vi "HeaderAction.vi"(0 "InstrClass":refnum<class "Agilent34410A.lvclass"> caption="DNL_LabVIEW Object in", 11 "error in (no error)":errorcluster caption="entrée d'erreur (pas d'erreur)") -> (4 "InstrClassOut":refnum<class "Agilent34410A.lvclass"> caption="DNL_LabVIEW Object out", 6 "DataNames":string[](array[string]), 8 "Instr Name":string, 10 "HeaderString":string, 13 "ArrDatNames":string[](array[string]), 14 "DisplayNames":string[](array[string]), 15 "error out":errorcluster caption="sortie d'erreur")   [LabVIEW 2019, in "Agilent34410A.lvclass"]
uses:
  Agilent34410A.lvclass
  C:/Programmes Labview/LabScanV1A/DevicesClass/BaseDevice/BaseDevice.lvclass
  Agilent34410A.lvclass/Agilent34410A.ctl
  BaseDevice/BaseDevice.lvclass
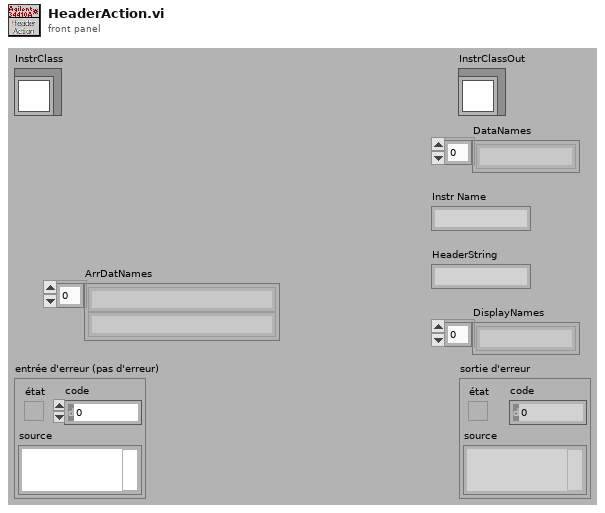
[diagram p1: front panel]
types:
  T1 = typedef "Agilent34410A.lvclass/Agilent34410A_Func.ctl" = enum16{"Read Function (Arb)", "Read Voltage (V)", "Read Current (A)", "Read 2W Resistance (Ohms)", "Read 4W Resistance (Ohms)"}
  T2 = typedef "Agilent34410A DMM_Func.ctl" = enum16{"Capacitance", "Continuity", "Current AC", "Current", "Diode", "Frequency", "4W Resistance", "Period", "Resistance", "Temperature", "Voltage AC", "Voltage"}
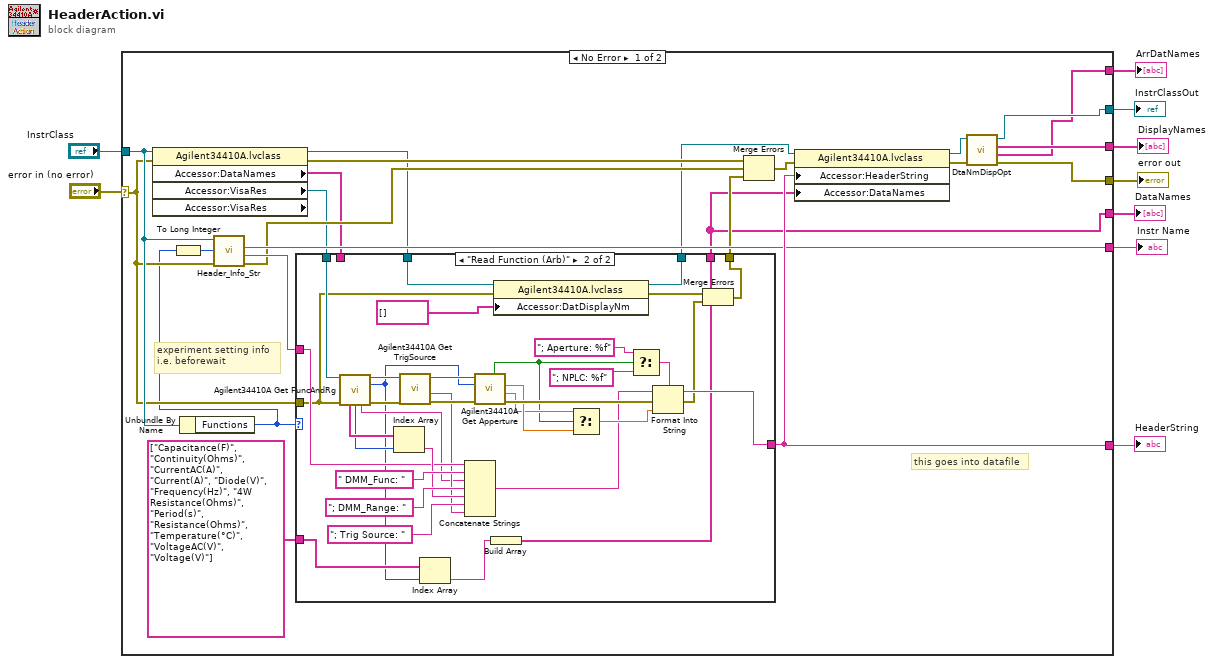
[diagram p0: block diagram]
diagram:
  n1 = case shown="No Error" "error in (no error)" {
    selector: "error in (no error)" -> [w21 w72]
    tunnel: [w31 _] -> w8
    tunnel: [w17 _] -> w7
    tunnel: "InstrClass" -> [w27 w73]
    tunnel: [w10 w72] -> w5
    tunnel: [w12 w73] -> w3
    tunnel: [w26 _] -> w4
    tunnel: [w28 _] -> w2
    tunnel: [w11 _] -> w1
    frame No Error {
      # "this goes into datafile"
      # "experiment setting info\ni.e. beforewait"
      n2 = property class="Agilent34410A.lvclass" props=["Accessor:DataNames", "Accessor:VisaRes", "Accessor:VisaRes"](reference=w27, error in=w21) -> (reference out=w16:refnum<class "Agilent34410A.lvclass">, error out=w32:errorcluster, "Accessor:DataNames"=w19:string[], "Accessor:VisaRes"=w22:refnum<visa-resource-name>)  [unwired: 1 out]
      n3 = Unbundle By Name(w27) -> ("Functions"=w13:T1)
      n4 = To Long Integer(number=w13) -> (32bit integer=w14:i32)
      n5 = call-dynamic "Header_Info_Str.vi"("error in (no error)"=w21, "Functions"=w14, "DefaultDev in"=w27) -> ("error out"=w23:errorcluster, "HdrInfoStr"=w25:string, "InstrumentName"=w26:string)  [unwired: 5 in, 1 out]
      n6 = case shown="\"Read Function (Arb)\"" w13 {
        tunnel: [w36 w50] -> w31
        tunnel: w25 -> [w36 w54]
        tunnel: w22 -> [_ w71]
        tunnel: w21 -> [w35 w42]
        tunnel: [w35 w39] -> w20
        tunnel: w19 -> [w34 _]
        tunnel: [w34 w38] -> w17
        tunnel: string[] ["Capacitance(F)", "Continuity(Ohms)", "CurrentAC(A)", "Current(A)", "Diode(V)", "Frequency(Hz)", "4W Resistance(Ohms)", "Period(s)", "Resistance(Ohms)", "Temperature(°C)", "VoltageAC(V)", "Voltage(V)"] ("Chaînes []") -> [_ w47]
        tunnel: w16 -> [w33 w44]
        tunnel: [w33 w43] -> w15
        frame Default {
        }
        frame "Read Function (Arb)" {
          n7 = call <userlib>:"Agilent34410A Get FuncAndRg.vi"("VISA Rsrc"=w71, "error in (no error)"=w42) -> ("VISA Rsrc Out"=w69:refnum<visa-resource-name>, "DMM Function"=w45:T2, "Function Ranges"=w70:string[], "Range Index"=w48:i32, "DMMFuncString"=w49:string, "error out"=w57:errorcluster)  [unwired: 5 in, 3 out]
          n8 = Index Array(array=w70, index=w48) -> (element=w55:string)
          n9 = call <userlib>:"Agilent34410A Get TrigSource.vi"("error in (no error)"=w57, "VISA Rsrc"=w69) -> ("error out"=w67:errorcluster, "TrigSrc String"=w52:string, "VISA Rsrc Out"=w68:refnum<visa-resource-name>)  [unwired: 5 in, 2 out]
          n10 = Index Array(array=w47, index=w45) -> (element=w46:string)
          n11 = Concatenate Strings(w54, " DMM_Func: " ("chaîne de format"), w49, "; DMM_Range: " ("chaîne de format"), w55, "; Trig Source: " ("chaîne de format"), w52) -> (w51:string)
          n12 = call <userlib>:"Agilent34410A Get Apperture.vi"("error in (no error)"=w67, "DMM Function"=w45, "VISA Rsrc"=w68) -> ("error out"=w66:errorcluster, "Aperture (s)"=w64:dbl, "NPLC Val"=w65:dbl, "Apperture Enable"=w61:bool)  [unwired: 2 in, 3 out]
          n13 = Build Array(w46) -> (w38:string[])
          n14 = property class="Agilent34410A.lvclass"(reference=w44, error in=w42, "Accessor:DatDisplayNm"=string[] [] ("DatDisplayNm")) -> (reference out=w43:refnum<class "Agilent34410A.lvclass">, error out=w40:errorcluster)
          n15 = Select(t=w64, s=w61, f=w65) -> (s? t:f=w60:dbl)
          n16 = Select(t="; Aperture: %f" ("chaîne de format"), s=w61, f="; NPLC: %f" ("chaîne de format")) -> (s? t:f=w59:string)
          n17 = Format Into String(format string=w59, initial string=w51, error in=w66, w60) -> (resulting string=w50:string, error out=w41:errorcluster)
          n18 = Merge Errors(w40, w41) -> (w39:errorcluster)
        }
      }
      n19 = Merge Errors(w32, w23, w20) -> (w24:errorcluster)
      n20 = property class="Agilent34410A.lvclass"(reference=w15, error in=w24, "Accessor:HeaderString"=w31, "Accessor:DataNames"=w17) -> (reference out=w29:refnum<class "Agilent34410A.lvclass">, error out=w30:errorcluster)
      n21 = call "DtaNmDispOpt.vi"("error in (no error)"=w30, "BaseDevice en entrée"=w29) -> ("error out"=w10:errorcluster, "ArrDisplayNames"=w11:string[], "DisplayNames"=w28:string[], "BaseDevice en sortie"=w12:refnum<class "Agilent34410A.lvclass">)  [unwired: 6 in]
    }
    frame Error {
    }
  }
  "error out" <- w5
  "InstrClassOut" <- w3
  "DataNames" <- w7
  "HeaderString" <- w8
  "Instr Name" <- w4
  "DisplayNames" <- w2
  "ArrDatNames" <- w1
